vi "defender normal.vi"(9 "balls":T1[](array[typedef]), 10 "IA State":T2={"our_robots"=[], "enemy_robots"=[], "balls"=[], "geometry"={"field_length"=0, "field_width"=0, "goal_width"=0, "goal_depth"=0, "center_circle_radius"=0, "defense_width"=0, "defense_depth"=0, "free_kick_from_defense_dist"=0, "penalty_spot_from_field_line_dist"=0, "penalty_line_from_spot_dist"=0, "half_moon_depth"=0, "half_moon_width"=0}, "IA Judge"={"stage"="", "command"="", "our_goalie_id"=0.0, "enemy_goalie_id"=0.0, "command enum"=enum."Halt", "Time"=enum."Azul"}, "Received Timestamp"=timestamp(0 s since 1904-01-01), "Events"={"Touch"=FALSE, "id touch"=0.0, "Ball out of \nVision"=FALSE, "Ball inside \nGoalie area"=FALSE, "Robot not responding"=FALSE, "Robots responding status"=[1.0, 1.0, 1.0, 1.0, 1.0, 1.0], "Enemy Ball \nPossession"=FALSE, "Id ini Possession"=0.0, "Ball Possesion"=FALSE, "Id Possesion"=0.0}}, 11 "Robot in":T3) -> (3 "Robot out":T3)   [LabVIEW 2017]
uses:
  Core/AI Robot.ctl
  Functions Enum.ctl
  AttackerStates.ctl
  Path Planning/RRT/PathDests.ctl
  Path Planning/RRT/PathDest.ctl
  Core/AI Input.ctl
  Core/AI Ball.ctl
  Core/Field Size.ctl
  Core/AI Judge.ctl
  Command Enum.ctl
  Util/Events/Events.ctl
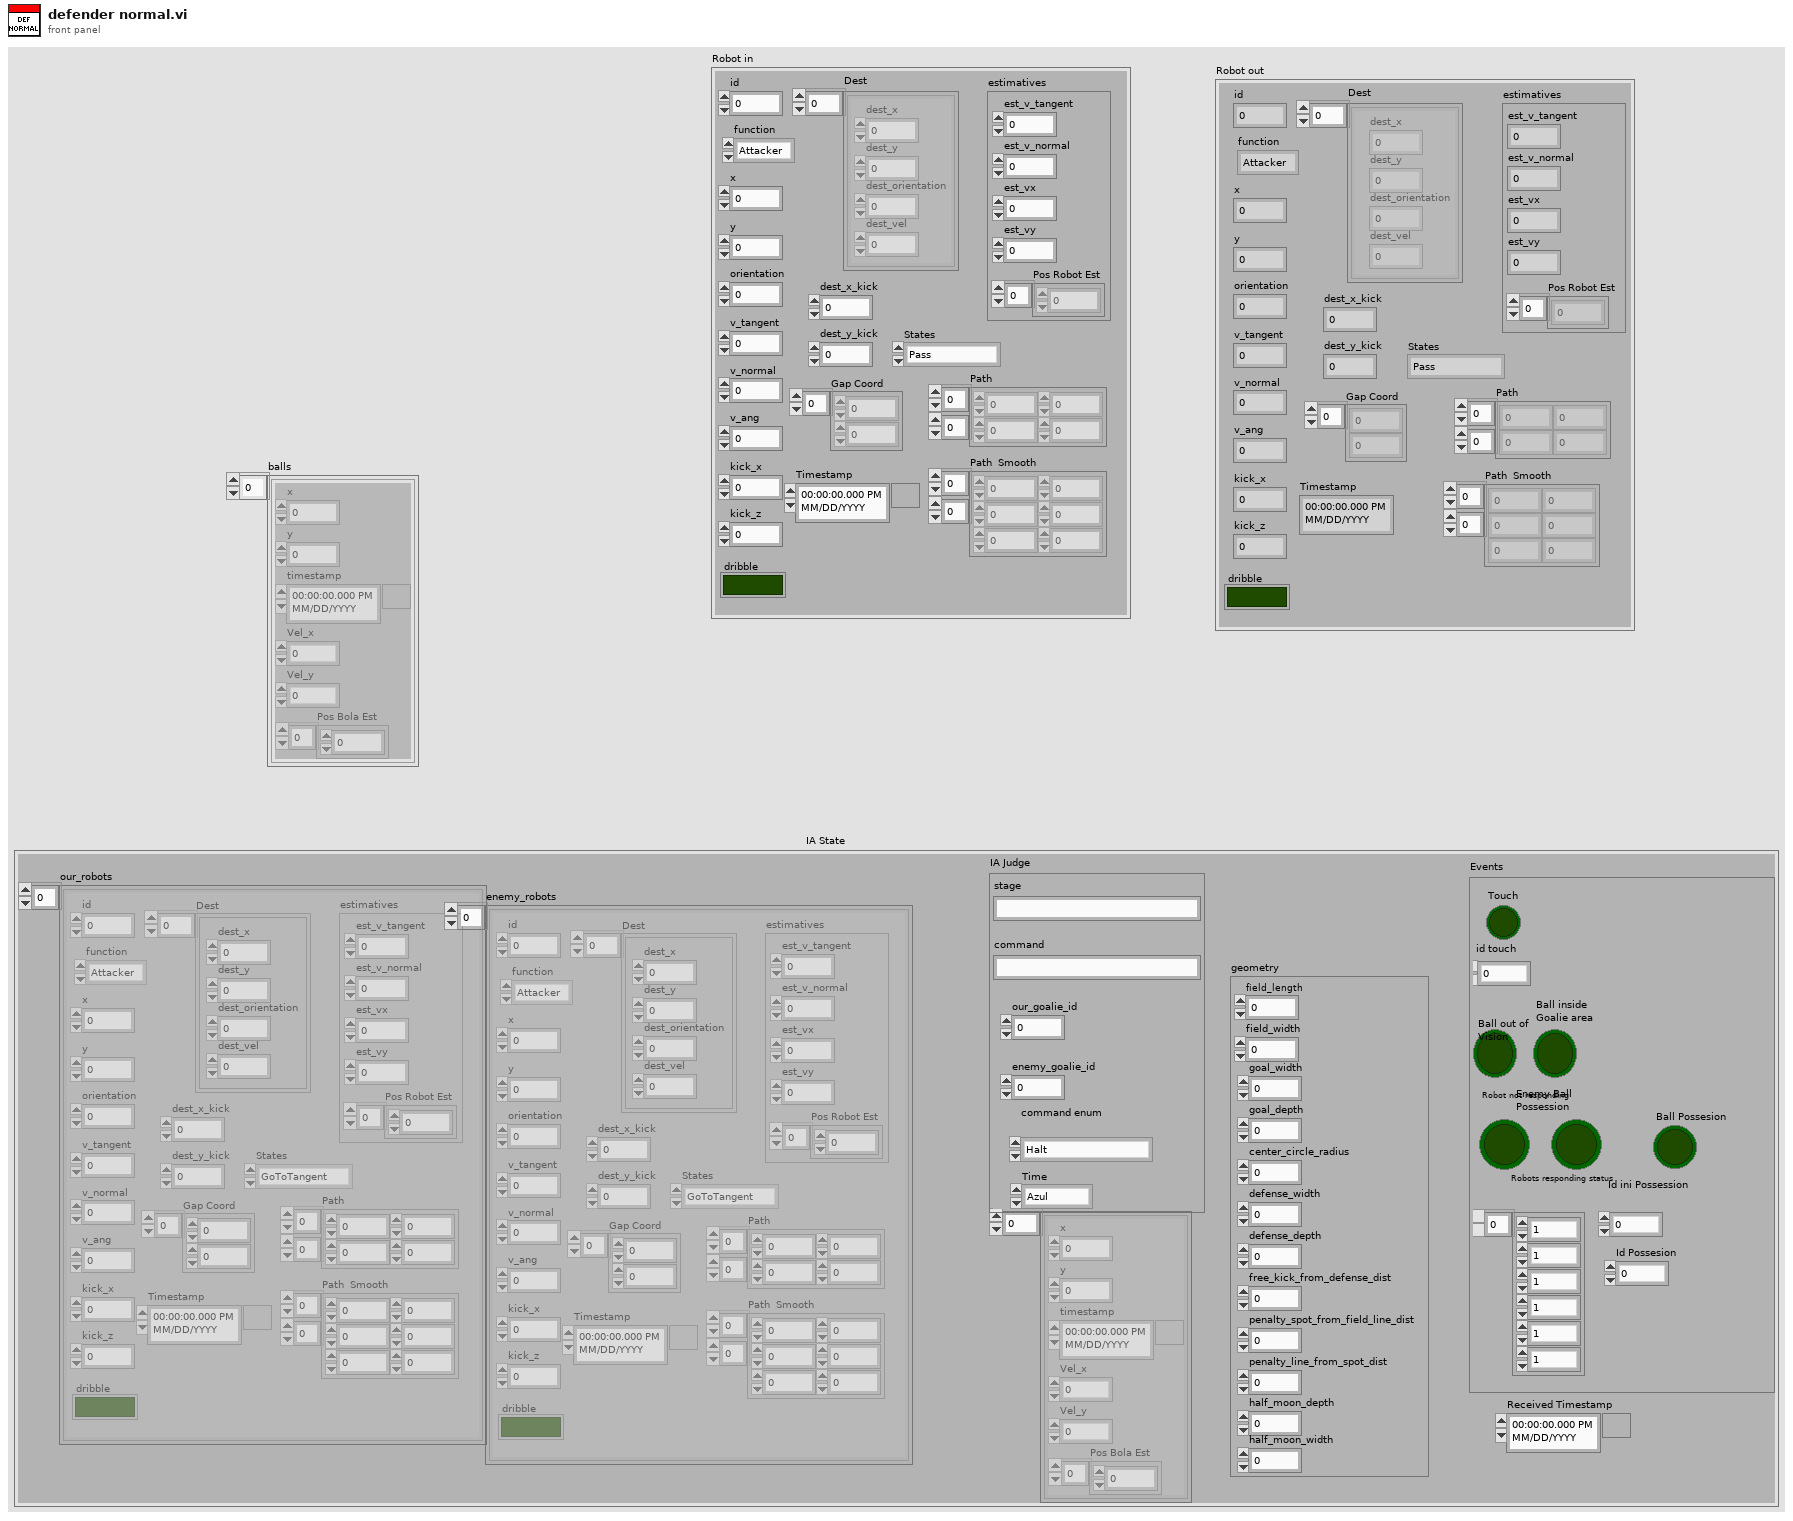
[diagram p1: front panel]
types:
  T1 = typedef "AI Ball.ctl" = cluster{"x":dbl, "y":dbl, "timestamp":timestamp, "Vel_x":dbl, "Vel_y":dbl, "Pos Bola Est":dbl[]}
  T2 = typedef "AI Input.ctl" = cluster{"our_robots":T3[], "enemy_robots":T3[], "balls":T1[], "geometry":T8, "IA Judge":T9, "Received Timestamp":timestamp, "Events":T11}
  T3 = typedef "AI Robot.ctl" = cluster{"id":u32, "function":T4, "x":dbl, "y":dbl, "orientation":dbl, "v_tangent":dbl, "v_normal":dbl, "v_ang":dbl, "kick_x":dbl, "kick_z":dbl, "dribble":bool, "Timestamp":timestamp, "estimatives":cluster{"est_v_tangent":dbl, "est_v_normal":dbl, "est_vx":dbl, "est_vy":dbl, "Pos Robot Est":dbl[]}, "dest_x_kick":dbl, "dest_y_kick":dbl, "Gap Coord":dbl[], "States":T5, "Path ":dbl[][], "Path  Smooth":dbl[][], "Dest":T6}
  T4 = typedef "Functions Enum.ctl" = enum16{"Attacker", "Goalie", "Defender", "Striker", "Goto 0", "Dummy", "Kicker", "ZigZag"}
  T5 = typedef "AttackerStates.ctl" = enum16{"Pass", "GoToTangent", "BallGetting", "GoToKick", ""}
  T6 = typedef "PathDests.ctl" = T7[]
  T7 = typedef "PathDest.ctl" = cluster{"dest_x":dbl, "dest_y":dbl, "dest_orientation":dbl, "dest_vel":dbl}
  T8 = typedef "Field Size.ctl" = cluster{"field_length":u32, "field_width":u32, "goal_width":u32, "goal_depth":u32, "center_circle_radius":u32, "defense_width":u32, "defense_depth":u32, "free_kick_from_defense_dist":u32, "penalty_spot_from_field_line_dist":u32, "penalty_line_from_spot_dist":u32, "half_moon_depth":u32, "half_moon_width":u32}
  T9 = typedef "AI Judge.ctl" = cluster{"stage":string, "command":string, "our_goalie_id":dbl, "enemy_goalie_id":dbl, "command enum":T10, "Time":enum16{"Azul", "Amarelo"}}
  T10 = typedef "Command Enum.ctl" = enum16{"Halt", "Stop", "Force Start", "PKA Normal Start", "Prepare Kickoff Ally", "PKE Normal Start", "Prepare Kickoff Enemy", "Prepare Penalty Ally", "PPA Normal Start", "Prepare Penalty Enemy", "PPE Normal Start", "Direct Free Enemy", "Direct Free Ally", "Indirect Free Enemy", "Indirect Free Ally", "Timeout Enemy", "Timeout Ally", "Goal Enemy", "Goal Ally", "Ball Placement Enemy", "Ball Placement Ally", "Normal Half Time", "Extra Time Break", "Extra Half Time", "None", "Post Game"}
  T11 = typedef "Events.ctl" = cluster{"Touch":bool, "id touch":dbl, "Ball out of \nVision":bool, "Ball inside \nGoalie area":bool, "Robot not responding":bool, "Robots responding status":dbl[], "Enemy Ball \nPossession":bool, "Id ini Possession":dbl, "Ball Possesion":bool, "Id Possesion":dbl}
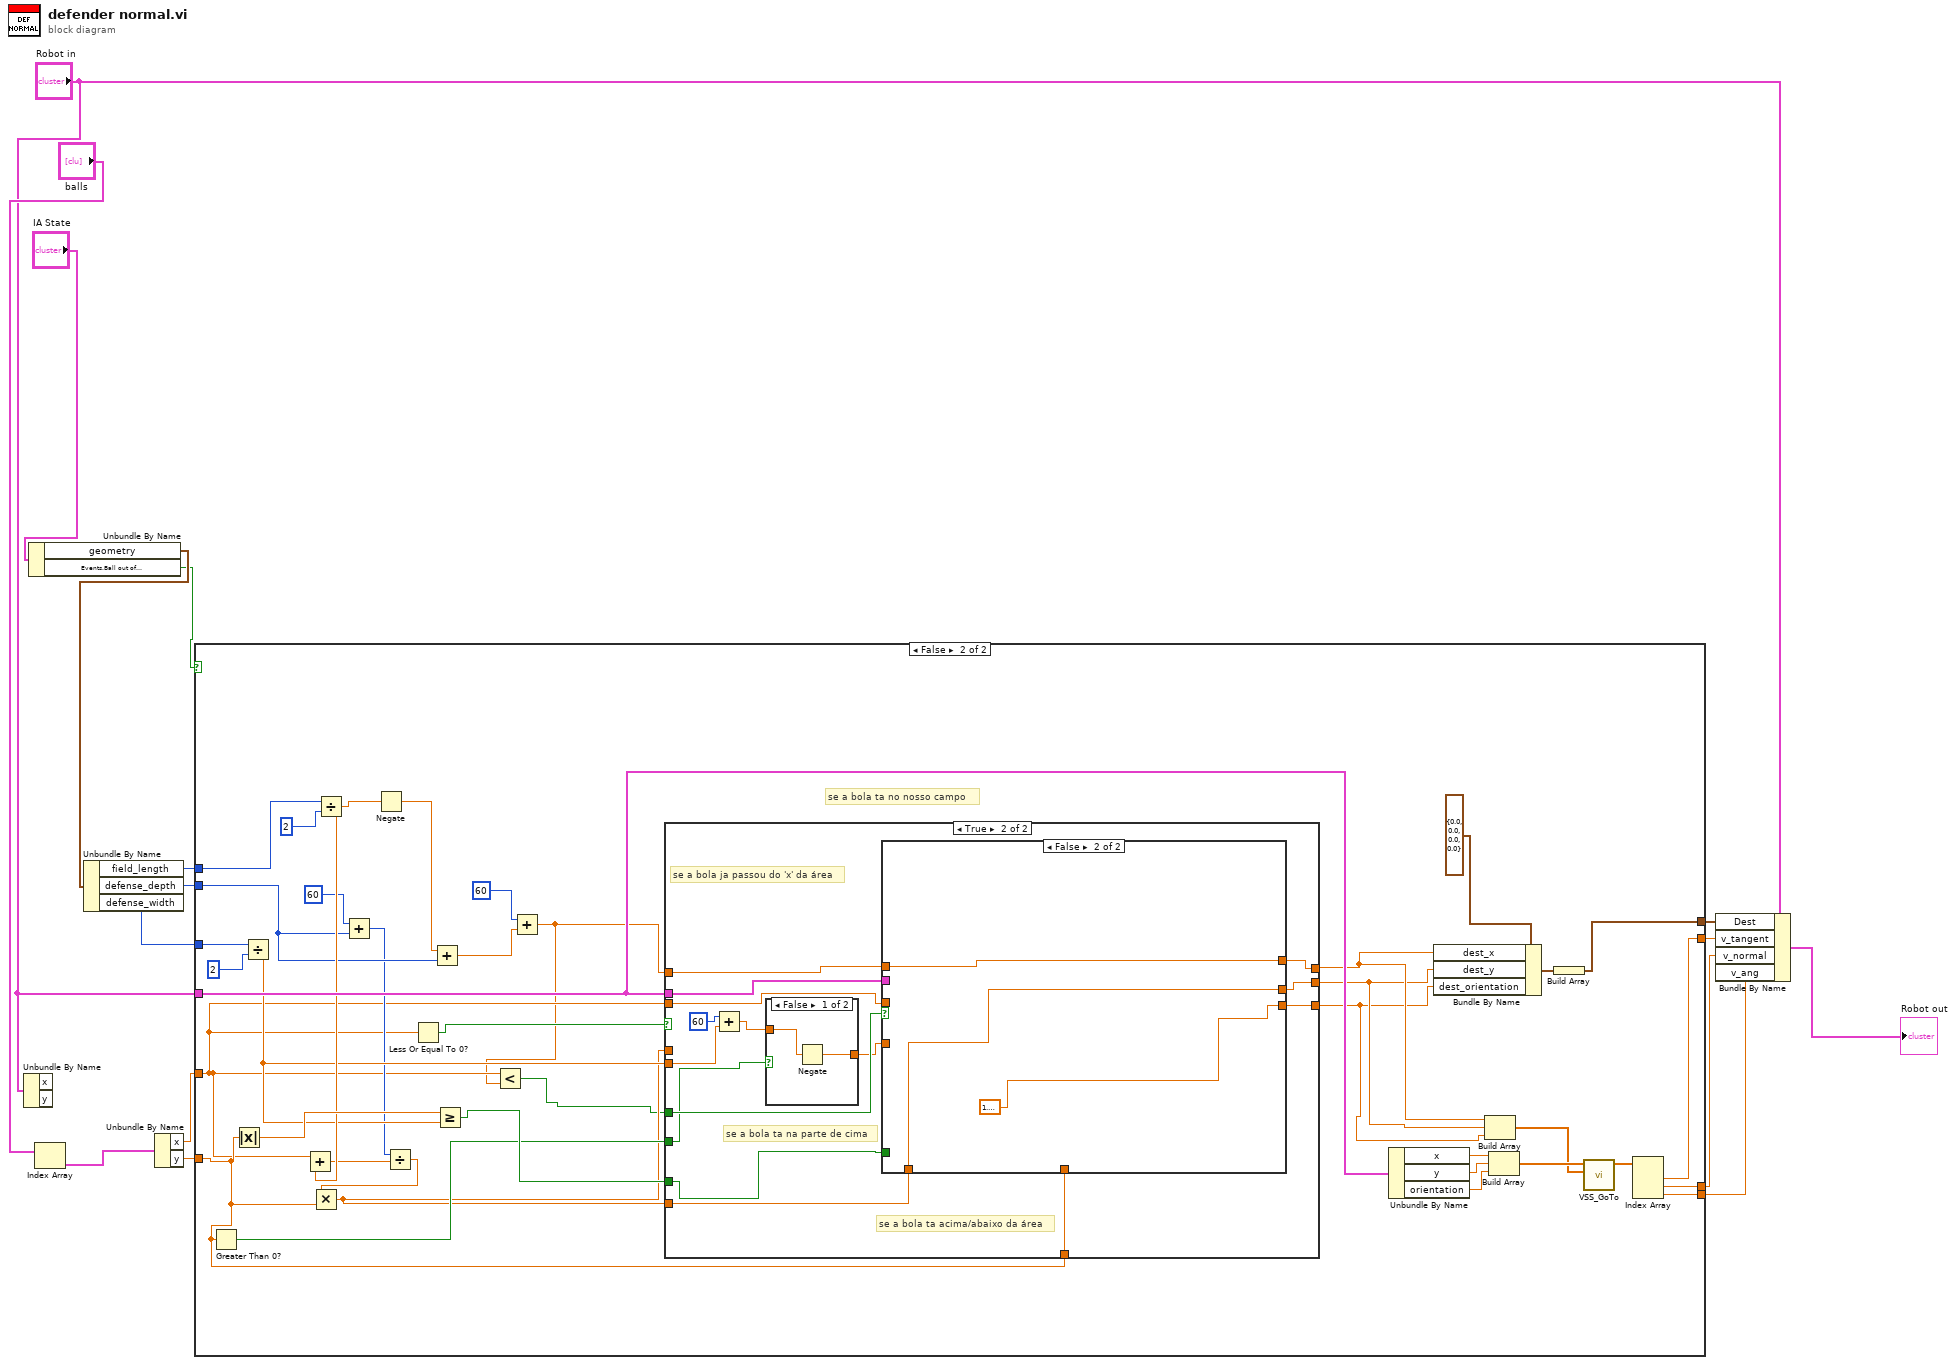
[diagram p0: block diagram]
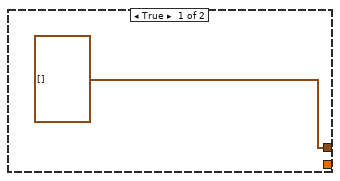
[diagram p2: hidden frame]
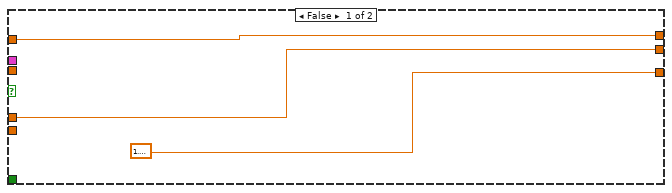
[diagram p3: hidden frame]
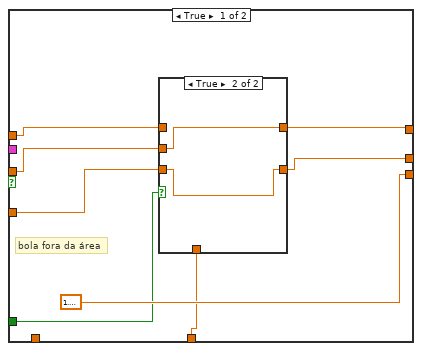
[diagram p5: hidden frame]
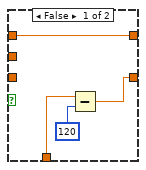
[diagram p6: hidden frame]
diagram:
  n1 = Unbundle By Name("Robot in") -> ()  [unwired: 2 out]
  n2 = Unbundle By Name("IA State") -> ("geometry"=w12:T8, "Events.Ball out of \nVision"=w1:bool)
  n3 = Index Array(array="balls") -> (element=w16:T1)  [unwired: 1 in]
  n4 = Unbundle By Name(w12) -> ("field_length"=w15:u32, "defense_depth"=w2:u32, "defense_width"=w11:u32)
  n5 = Unbundle By Name(w16) -> ("x"=w3:dbl, "y"=w4:dbl)
  n6 = case shown="False" w1 {
    tunnel: w15 -> [_ w55]
    tunnel: w11 -> [_ w51]
    tunnel: [T7[] [] w42] -> w10
    tunnel: "Robot in" -> [_ w39]
    tunnel: [_ w35] -> w7
    tunnel: [_ w34] -> w6
    tunnel: [_ w33] -> w5
    tunnel: w4 -> [_ w22]
    tunnel: w3 -> [_ w20]
    tunnel: w2 -> [_ w24]
    frame True {
    }
    frame False {
      # "se a bola ta no nosso campo"
      n7 = Greater Than 0?(x=w22) -> (x > 0?=w30:bool)
      n8 = Absolute Value(x=w22) -> (abs(x)=w54:dbl)
      n9 = Divide(x=w51, y=2) -> (x/y=w26:dbl)
      n10 = Divide(x=w55, y=2) -> (x/y=w28:dbl)
      n11 = Add(x=w20, y=w28) -> (x+y=w27:dbl)
      n12 = Add(x=60, y=w24) -> (x+y=w23:u32)
      n13 = Negate(x=w28) -> (-x=w53:dbl)
      n14 = Divide(x=w23, y=w27) -> (x/y=w50:dbl)
      n15 = Multiply(x=w50, y=w22) -> (x*y=w21:dbl)
      n16 = Less Or Equal To 0?(x=w20) -> (x <= 0?=w29:bool)
      n17 = Add(x=w53, y=w24) -> (x+y=w31:dbl)
      n18 = Greater Or Equal?(x=w54, y=w26) -> (x >= y?=w49:bool)
      n19 = Add(x=60, y=w31) -> (x+y=w19:dbl)
      n20 = Less?(x=w20, y=w19) -> (x < y?=w18:bool)
      n21 = case shown="True" w29 {
        tunnel: w39 -> [_ w74]
        tunnel: w19 -> [w59 w73]
        tunnel: w18 -> [_ w72]
        tunnel: w30 -> [_ w71]
        tunnel: w26 -> [_ w64]
        tunnel: w20 -> [_ w70]
        tunnel: w21 -> [w58 _]
        tunnel: w49 -> [_ w62]
        tunnel: [w59 w69] -> w38
        tunnel: [w58 w68] -> w37
        tunnel: [1.5707963267948966 w67] -> w36
        tunnel: w22 -> [_ w63]
        tunnel: w21 -> [_ w60]
        frame False {
        }
        frame True {
          # "se a bola ta acima/abaixo da área"
          # "se a bola ja passou do 'x' da área"
          # "se a bola ta na parte de cima"
          n22 = Add(x=60, y=w64) -> (x+y=w66:dbl)
          n23 = case shown="False" w71 {
            tunnel: w66 -> [w76 w77]
            tunnel: [w75 w77] -> w61
            frame False {
              n24 = Negate(x=w76) -> (-x=w75:dbl)
            }
            frame True {
            }
          }
          n25 = case shown="False" w72 {
            tunnel: w74 -> [_ _]
            tunnel: w61 -> [w81 _]
            tunnel: w73 -> [w80 w94]
            tunnel: w70 -> [w78 _]
            tunnel: [w79 w94] -> w69
            tunnel: [w84 w92] -> w68
            tunnel: [1.5707963267948966 1.5707963267948966] -> w67
            tunnel: w62 -> [w82 _]
            tunnel: w63 -> [w83 _]
            tunnel: w60 -> [_ w92]
            frame True {
              # "bola fora da área"
              n26 = case shown="True" w82 {
                tunnel: w81 -> [_ w91]
                tunnel: [w86 w91] -> w84
                tunnel: w83 -> [w88 _]
                tunnel: w80 -> [w89 _]
                tunnel: [w89 w90] -> w79
                tunnel: w78 -> [_ w90]
                frame False {
                  n27 = Subtract(x=w88, y=120) -> (x-y=w86:dbl)
                }
                frame True {
                }
              }
            }
            frame False {
            }
          }
        }
      }
      n28 = Unbundle By Name(w39) -> ("x"=w45:dbl, "y"=w48:dbl, "orientation"=w47:dbl)
      n29 = Bundle By Name(cluster=T7 {"dest_x"=0.0, "dest_y"=0.0, "dest_orientation"=0.0, "dest_vel"=0.0} ("element"), "dest_x"=w38, "dest_y"=w37, "dest_orientation"=w36) -> (w41:T7)
      n30 = Build Array(w38, w37, w36) -> (w44:dbl[])
      n31 = Build Array(w45, w48, w47) -> (w46:dbl[])
      n32 = Build Array(w41) -> (w42:T7[])
      n33 = call "VSS_GoTo.vi"("SetPoint"=w44, "Position"=w46) -> ("Output Vel"=w43:dbl[])  [unwired: 9 in]
      n34 = Index Array(array=w43) -> (element #1=w35:dbl, element #2=w34:dbl, element #3=w33:dbl)  [unwired: 3 in]
    }
  }
  n35 = Bundle By Name(cluster="Robot in", "Dest"=w10, "v_tangent"=w7, "v_normal"=w6, "v_ang"=w5) -> (→"Robot out":T3)
